vi "EventLog.SourceBuffer.vi"(7 "Action":T5=enum."get", 8 "error in (no error)":errorcluster, 10 "Event in":T1={"ts"=0.0, "lev"=enum."Debug", "usr"=0, "src"=enum."All", "msg"=enum."Log out", "arg"=[], "msg_str"=""} {"ts" format="%<%X\n%x>T"}) -> (0 "error out":errorcluster, 1 "changed?/unconfirmed?":bool, 2 "Events":T1[](array[typedef]) {"ts" format="%<%X\n%x>T"})   [LabVIEW 2013]
uses:
  EventLog.SourceBuffer.Action.ctl
  EventLog.EventGui.ctl
  EventLog.EventLevel.ctl
  EventLog.EventSource.ctl
  Translator/Translator.Message.ctl
panel:
  out "All Events":T1[](array[typedef]) {"ts" format="%<%X\n%x>T"}
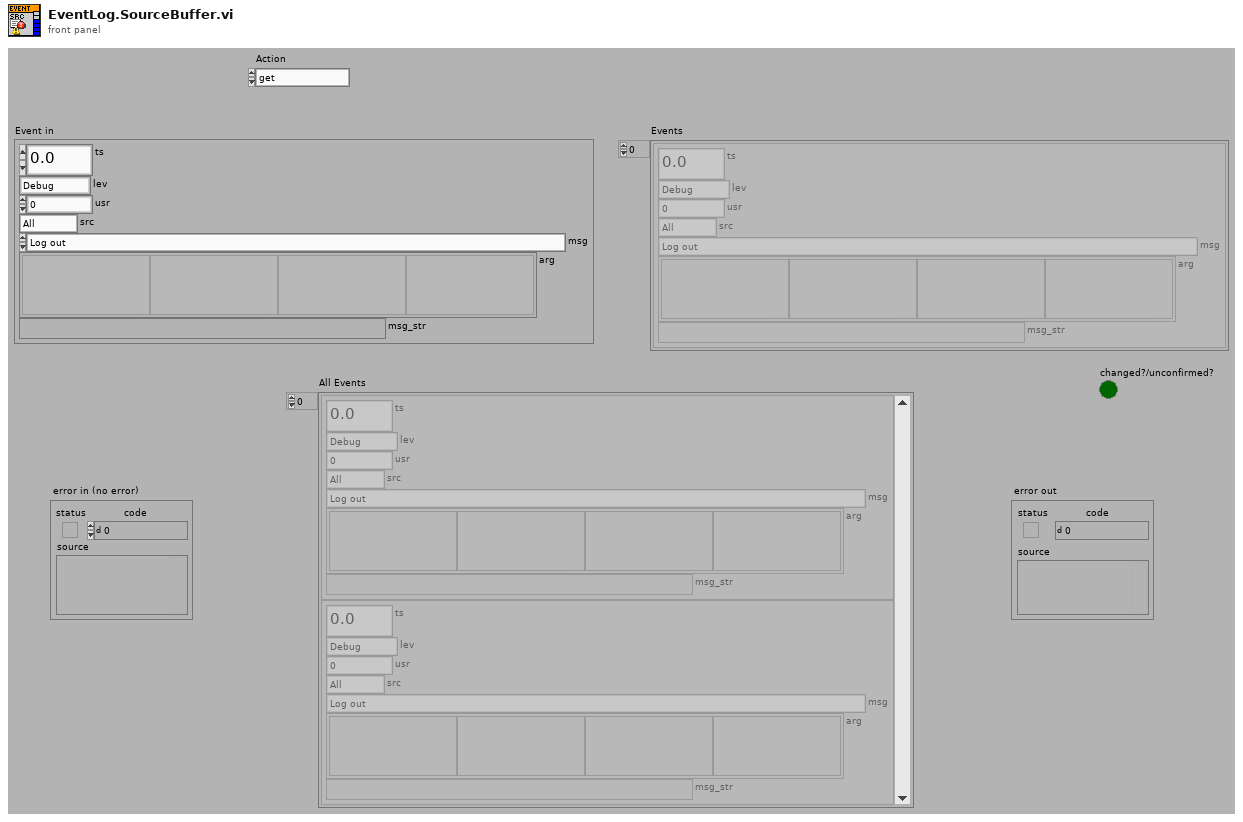
[diagram p1: front panel]
types:
  T1 = typedef "EventLog.EventGui.ctl" = cluster{"ts":dbl, "lev":T2, "usr":i32, "src":T3, "msg":T4, "arg":variant[], "msg_str":string}
  T2 = typedef "EventLog.EventLevel.ctl" = enum8{"Debug", "Info", "Warning", "Error"}
  T3 = typedef "EventLog.EventSource.ctl" = enum16{"All", "Gui", "DB", "Seq", "File", "DIO", "AI", "AO", "IFM", "CPX"}
  T4 = typedef "Translator.Message.ctl" = enum16{"-", "Event confirmed", "Log out", "Log in", "Shutdown", "Cancel", "Start", "Error %d >> %s", "Error %d >> %s >> %s", "Starting %s", "Quitting %s", "User %s level %s added", "User %s level %s deleted", "User %s level %s changed to %s", "Configured", "Initializing", "Quitting", "Loading", "Running", "Stopped", "Do you want to continue?", "Calibration", "Log out?", "System", "All", "IDLE", "Translating...%s", "Not found", "Alarm %s", "Restart is required to translate the application! Do you want to restart the PC?", "Restart cancelled. Be aware that some controls may not be fully translated until you restart the application.", "New version available!", "The software is up-to-date", "PC software will be updated after rebooting the PC. Do you want to reboot now?", "RT software will be updated. Make sure that no process is running. Do you want to reboot RT now?", "Updating RT firmware. Please wait...", "Update failed: %s", "Rebooting...", "Rebooting RT. Please wait...", "RT updated to version %s", "Timeout error during update. Check if RT is working", "Run", "Skip", "Abort", "Please wait...", "Put reference number...", "Folder '%s' is missing", "File '%s' is missing", "File '%s' is broken", "File '%s' is running", "Log file '%s' started", "Step '%s' added to log file", "Log file '%s' ended", "Test steps are missing", "Output %s = %.3f"}
  T5 = typedef "EventLog.SourceBuffer.Action.ctl" = enum16{"init", "new", "confirm", "check", "get", "get alarms"}
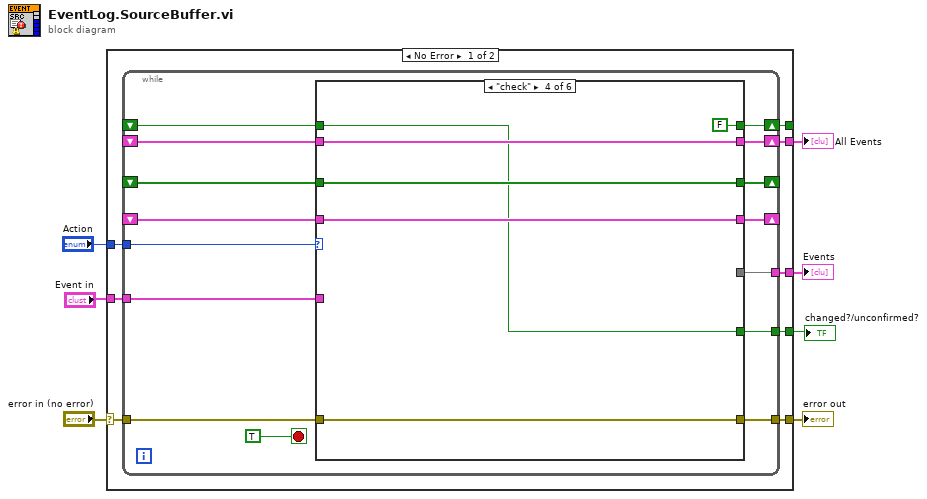
[diagram p0: block diagram]
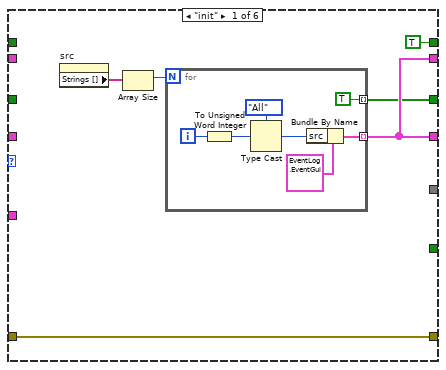
[diagram p2: hidden frame]
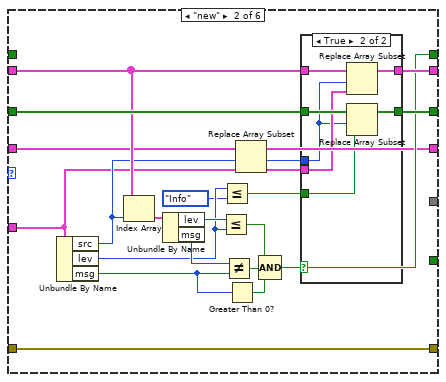
[diagram p3: hidden frame]
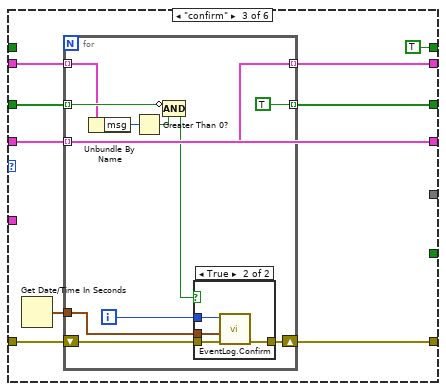
[diagram p5: hidden frame]
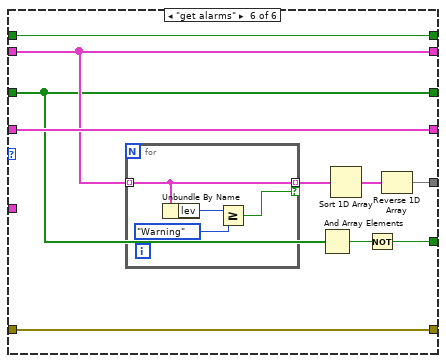
[diagram p8: hidden frame]
diagram:
  n1 = case shown="No Error" "error in (no error)" {
    selector: "error in (no error)" -> [w15 w123]
    tunnel: [w12 w123] -> w6
    tunnel: "Action" -> [w14 _]
    tunnel: "Event in" -> [w13 _]
    tunnel: [w11 _] -> w4
    tunnel: [w10 _] -> _
    tunnel: [w9 _] -> w2
    tunnel: [w8 _] -> w1
    frame No Error {
      n2 = while {
        tunnel: w15 -> [w25]
        tunnel: w14 -> [w30]
        tunnel: w13 -> [w29]
        shift-right: [w28] -> w9
        shift-left: _ -> [w27]
        tunnel: [w24] -> w12
        shift-right: [w23] -> _
        shift-left: _ -> [w22]
        shift-right: [w21] -> _
        shift-left: _ -> [w20]
        tunnel: [w19] -> w11
        shift-right: [w18] -> w10
        shift-left: _ -> [w17]
        tunnel: [w16] -> w8
        stop <- TRUE stop-if-true
        n3 = case shown="\"check\"" w30 {
          tunnel: w29 -> [_ w45 _ _ _ _]
          tunnel: [w34 w63 w75 w99 w105 w116] -> w28
          tunnel: w27 -> [_ w60 w80 w99 w105 w116]
          tunnel: w25 -> [w36 w59 w78 w103 w108 w118]
          tunnel: [w36 w59 w74 w103 w108 w118] -> w24
          tunnel: [w34 w44 w76 w102 w107 w117] -> w23
          tunnel: w22 -> [_ w46 w76 w102 w107 w117]
          tunnel: [w33 w61 w77 w101 w106 w111] -> w21
          tunnel: w20 -> [_ w62 w81 w101 w106 w111]
          tunnel: [_ _ _ _ w105 w112] -> w19
          tunnel: [TRUE w53 TRUE FALSE w104 w114] -> w18
          tunnel: w17 -> [_ _ _ w98 w104 w114]
          tunnel: [_ _ _ w98 w104 w109] -> w16
          frame "init" {
            n4 = property on="src" class="Enum (strict)"() -> ("Strings []"=w31:string[])  [unwired: 2 in, 2 out]
            n5 = Array Size(array=w31) -> (size(s)=w35:i32)
            n6 = for {
              N: w35 -> [_]
              tunnel: [w38] -> w34 mode=indexing
              tunnel: [TRUE] -> w33 mode=indexing
              i -> [w41]
              n7 = To Unsigned Word Integer(number=w41) -> (unsigned 16bit integer=w40:u16)
              n8 = Type Cast(type=EventLog.EventSource."All" ("group"), x=w40) -> (*(type *) &x=w42:T3)
              n9 = Bundle By Name(cluster=T1 {"ts"=0.0, "lev"=enum."Debug", "usr"=0, "src"=enum."All", "msg"=enum."-", "arg"=[], "msg_str"=""} ("Event in"), "src"=w42) -> (w38:T1)
            }
          }
          frame "new" {
            n10 = Unbundle By Name(w45) -> ("src"=w47:T3, "lev"=w50:T2, "msg"=w52:T4)
            n11 = Index Array(array=w60, index=w47) -> (element=w58:T1)
            n12 = Unbundle By Name(w58) -> ("lev"=w57:T2, "msg"=w56:T4)
            n13 = Less Or Equal?(x=w57, y=w50) -> (x <= y?=w55:bool)
            n14 = Less Or Equal?(x=w50, y=EventLog.EventLevel."Info") -> (x <= y?=w48:bool)
            n15 = Not Equal?(x=w56, y=w52) -> (x != y?=w54:bool)
            n16 = Greater Than 0?(x=w52) -> (x > 0?=w51:bool)
            n17 = Replace Array Subset(array=w46, new element=w45, index=w47) -> (w44:T1[])
            n18 = Compound Arithmetic op=AND(w55, w54, w51) -> (w53:bool)
            n19 = case shown="True" w53 {
              tunnel: [w65 w72] -> w63
              tunnel: w62 -> [w64 w71]
              tunnel: [w64 w70] -> w61
              tunnel: w60 -> [w65 w69]
              tunnel: w45 -> [_ w68]
              tunnel: w47 -> [_ w67]
              tunnel: w48 -> [_ w66]
              frame False {
              }
              frame True {
                n20 = Replace Array Subset(array=w69, new element=w68, index=w67) -> (w72:T1[])
                n21 = Replace Array Subset(array=w71, new element=w66, index=w67) -> (w70:bool[])
              }
            }
          }
          frame "confirm" {
            n22 = Get Date/Time In Seconds() -> (seconds since 1Jan1904=w79:timestamp)
            n23 = for {
              tunnel: w81 -> [w90] mode=indexing
              tunnel: w80 -> [w89] mode=indexing
              tunnel: w79 -> [w85]
              tunnel: [TRUE] -> w77 mode=indexing
              tunnel: w76 -> [w83] mode=indexing
              tunnel: [w83] -> w75 mode=indexing
              shift-right: [w86] -> w74
              shift-left: w78 -> [w88]
              i -> [w82]
              n24 = Unbundle By Name(w89) -> ("msg"=w92:T4)
              n25 = Greater Than 0?(x=w92) -> (x > 0?=w91:bool)
              n26 = Compound Arithmetic op=AND(invert w90, w91) -> (w87:bool)
              n27 = case shown="True" w87 {
                tunnel: w88 -> [w93 w97]
                tunnel: [w93 w96] -> w86
                tunnel: w85 -> [_ w95]
                tunnel: w82 -> [_ w94]
                frame False {
                }
                frame True {
                  n28 = call "EventLog.Confirm.vi"("error in"=w97, "current time"=w95, "src"=w94) -> ("error out"=w96:errorcluster)  [unwired: 8 in]
                }
              }
            }
          }
          frame "check" {
          }
          frame "get" {
          }
          frame "get alarms" {
            n29 = for {
              tunnel: w116 -> [w120] mode=indexing
              tunnel: [w120] -> w115 mode=indexing if=w119
              n30 = Unbundle By Name(w120) -> ("lev"=w122:T2)
              n31 = Greater Or Equal?(x=w122, y=EventLog.EventLevel."Warning" ("x")) -> (x >= y?=w119:bool)
            }
            n32 = And Array Elements(Boolean array=w111) -> (logical AND=w110:bool)
            n33 = Sort 1D Array(array=w115) -> (sorted array=w113:T1[])
            n34 = Not(x=w110) -> (.not. x?=w109:bool)
            n35 = Reverse 1D Array(array=w113) -> (reversed array=w112:T1[])
          }
        }
      }
    }
    frame Error {
    }
  }
  "error out" <- w6
  "Events" <- w4
  "changed?/unconfirmed?" <- w1
  "All Events" <- w2
